vi "Get Server Stats.vi"(8 "error in (no error)":errorcluster, 11 "Connection ID":refnum<k5>) -> (0 "error out":errorcluster, 1 "Server stats":T1={"scan rate"=10.0, "# connections"=0, "channel settings"=[]} {"channel settings"."lower input limits" format="%.4f"; "channel settings"."upper input limits" format="%.4f"; "scan rate" format="%.2f"}, 2 "bytes read":i32, 3 "Connection ID":refnum<k5>)   [LabVIEW 2012]
uses:
  DataServer/Server stats.ctl
  DataServer/Server Stats.vi
panel:
  # "Hz"
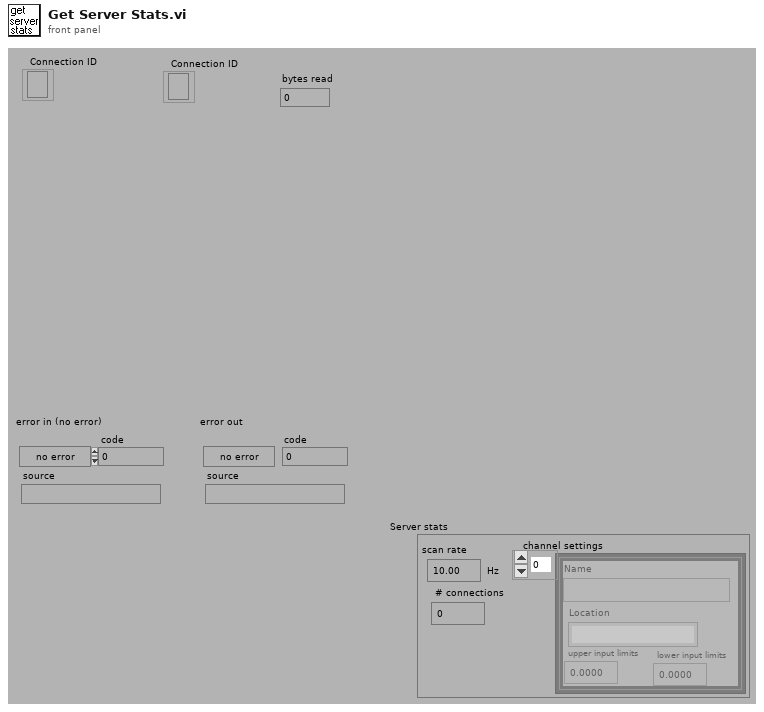
[diagram p1: front panel]
types:
  T1 = typedef "Server stats.ctl" = cluster{"scan rate":dbl, "# connections":i32, "channel settings":cluster{"Name":string, "upper input limits":sgl, "lower input limits":sgl, "Location":string}[]}
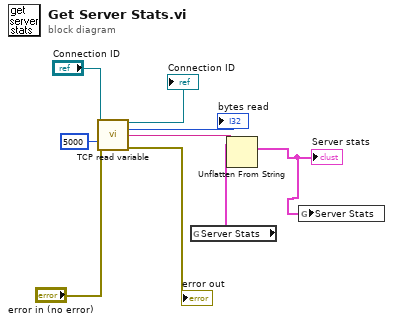
[diagram p0: block diagram]
diagram:
  n1 = call "TCP read variable.vi"("connection ID"="Connection ID", "timeout ms (25000)"=5000, "error in (no error)"="error in (no error)") -> ("connection ID out"=→"Connection ID":refnum<k5>, "bytes read"=→"bytes read":i32, "data out"=w4:string, "error out"=→"error out":errorcluster)  [unwired: 9 in]
  n2 = global read "Server Stats.vi" "Server Stats"() -> (w2:T1)
  n3 = Unflatten From String(type=w2, binary string=w4) -> (value=w1:T1)  [unwired: 3 in, 2 out]
  "Server stats" <- w1
  n4 = global write "Server Stats.vi" "Server Stats"(w1) -> ()
